vi "BRig_dataCurrent_iSpout.vi"() -> (2 "output_iSpout":i32)   [LabVIEW 2014]
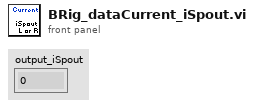
[diagram p1: front panel]
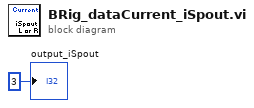
[diagram p0: block diagram]
diagram:
  "output_iSpout" <- 3 ("output_iBlock")
